vi "Close BLE Server.vi"(8 "Error In":errorcluster) -> (0 "Error Out":errorcluster)   [LabVIEW 2016]
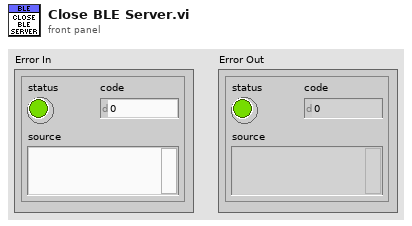
[diagram p1: front panel]
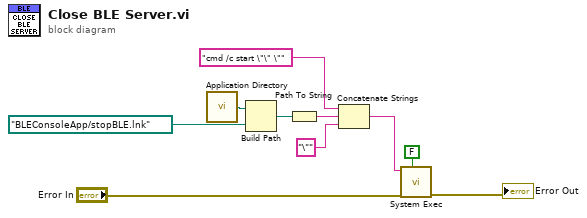
[diagram p0: block diagram]
diagram:
  n1 = call <vilib>:"Application Directory.vi"() -> ("Application Directory"=w10:path)
  n2 = Build Path(base path=w10, name or relative path=path "BLEConsoleApp/stopBLE.lnk") -> (appended path=w8:path)
  n3 = Path To String(path=w8) -> (string=w6:string)
  n4 = Concatenate Strings("cmd /c start \"\" \"" ("string"), w6, "\"" ("string")) -> (w5:string)
  n5 = call <vilib>:"System Exec.vi"("wait until completion? (T)"=FALSE, "error in (no error)"="Error In", "command line"=w5) -> ("error out"=→"Error Out":errorcluster)  [unwired: 5 in, 3 out]
